vi "testmatlab2.vi"   [LabVIEW 2020]
uses:
  <vilib>/Platform/storage/Storage.llb/usiSequenceRepresentation.ctl
  <vilib>/Platform/storage/Storage.llb/usiOverwriteOptions.ctl
  <vilib>/Platform/storage/lvStorage.llb/_openStorageWithRootAutoDetect.vi
  <vilib>/Platform/storage/lvStorage.llb/xStorage/xStorageSupp/ErrorOut.vi
  <vilib>/Platform/storage/Storage.llb/_createExplicitChildObject.vi
  <vilib>/Platform/storage/Storage.llb/__savePropString.vi
  <vilib>/Platform/storage/lvStorage.llb/_saveFloat64Channel.vi
  <vilib>/Platform/storage/Storage.llb/Get Object Info.vi
  <vilib>/Platform/storage/Storage.llb/__closeStorageFromObject.vi
  <vilib>/Platform/storage/lvStorage.llb/xStorage/Open Data Storage/Open Data Storage.xnode
  <vilib>/Platform/storage/lvStorage.llb/xStorage/Write Data/Write Data.xnode
  <vilib>/Platform/storage/lvStorage.llb/xStorage/Close Data Storage/Close Data Storage.xnode
types:
  T1 = enum16{"open", "open or create", "create or replace", "create", "open (read only)"}
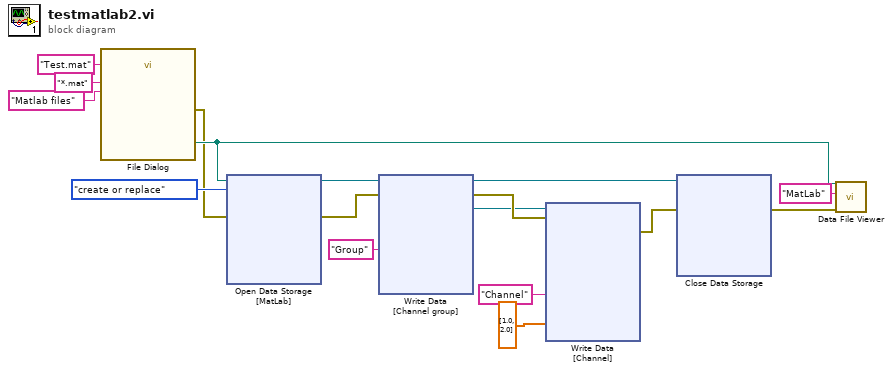
[diagram p0: block diagram]
diagram:
  n1 = call "File Dialog"("default name"="Test.mat", "pattern (all files)"="*.mat", "pattern label"="Matlab files") -> ("selected path"=w7:path, "error out"=w3:errorcluster)  [unwired: 9 in, 2 out]
  n2 = xnode "Open Data Storage\n[MatLab]"("file path"=w7, "function (open:0)"=T1."create or replace", "error in (no error)"=w3) -> ("storage refnum (file)"=w12:refnum<k20>, "error out"=w11:errorcluster)  [unwired: 2 in, 1 out]
  n3 = xnode ("Write Data\n[Channel group]")("Name"="Group", "storage refnum (file)"=w12, "error in"=w11) -> ("storage refnum (file) out"=w2:refnum<k20>, "error out"=w10:errorcluster, "storage refnum (channel group)"=w8:refnum<k20>)
  n4 = xnode "Write Data\n[Channel]"("Name"="Channel", "Signal"=dbl[] [1.0, 2.0], "storage refnum (channel group)"=w8, "error in"=w10) -> ("error out"=w1:errorcluster)  [unwired: 2 in, 2 out]
  n5 = xnode "Close Data Storage\n"("storage refnum (file)"=w2, "error in (no error)"=w1) -> ("error out"=w15:errorcluster)  [unwired: 1 out]
  n6 = call <vilib>:"Data File Viewer.vi"("error in (no error)"=w15, "DataPlugin name"="MatLab", "file path"=w7) -> ()  [unwired: 2 in, 3 out]
